vi "Dynamic Generation of Formula for Vtip.vi"(11 "Voltage (V)":T1={"Schedule"=enum."Constant", "Settings"=variant(dbl 10.0)}) -> (3 "Voltage (V) 2":T1={"Schedule"=enum."Constant", "Settings"=variant(dbl 10.0)})   [LabVIEW 2019]
uses:
  typedefs/Voltage - cluster.ctl
  typedefs/Schedule - enum.ctl
  typedefs/Schedule Types/Schedule--Formula.ctl
  <vilib>/gmath/NI_Gmath.lvlib
panel:
  out "error":i32
  in  "formula":string="1*(step(170-t)*cos(0.62831853071*t)+step(t-170)*cos(0.62831853071*(t-170))*(-1))"
  out "XY Graph":cluster{"X Values":dbl[], "Y Values":dbl[]}(graph)
  in  "Resolution (nm)":dbl=0.001
  in  "Length (nm)":dbl=340.0
  in  "OK":bool
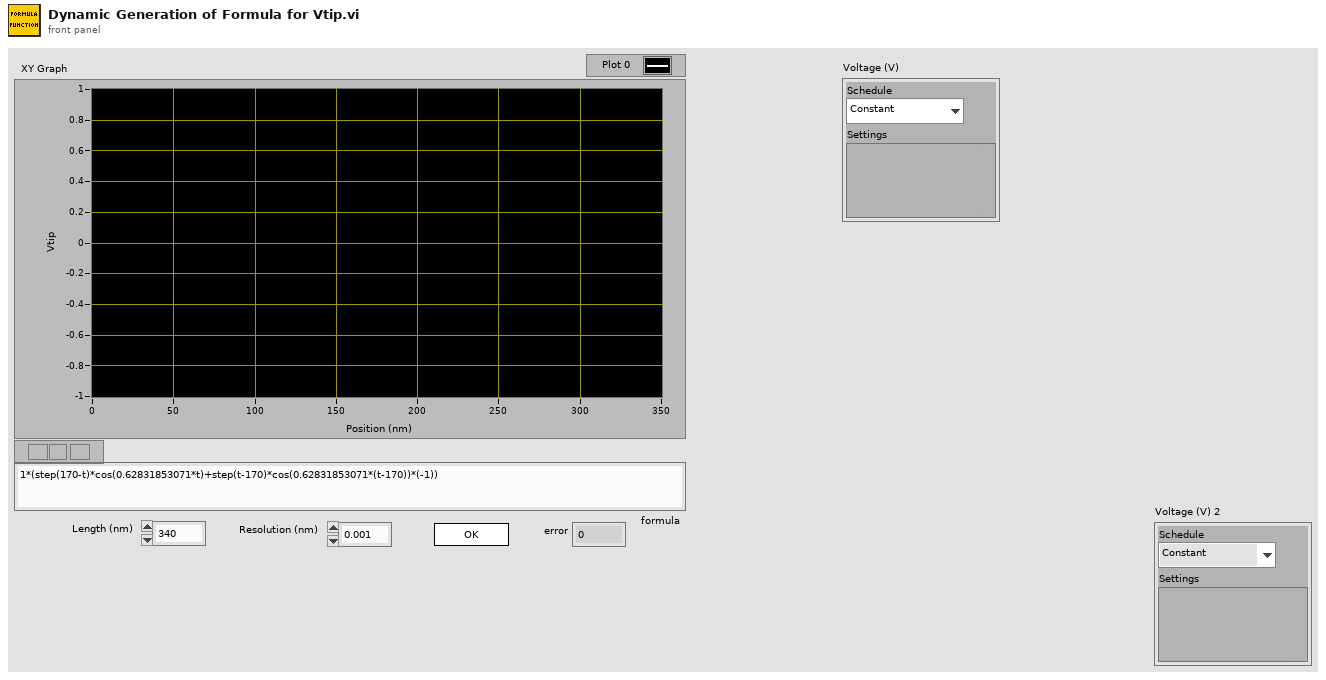
[diagram p1: front panel]
types:
  T1 = typedef "Voltage - cluster.ctl" = cluster{"Schedule":T2, "Settings":variant}
  T2 = typedef "Schedule - enum.ctl" = enum16{"Constant", "Ramp", "Fn. Generator", "Formula"}
  T3 = enum32{"invalid app kind", "Development System", "Run Time System", "Student Edition", "Embedded LabVIEW", "Evaluation", "Custom"}
  T4 = enum32{"Invalid", "Standard", "Closed", "Hidden", "Minimized", "Maximized"}
  T5 = typedef "Schedule--Formula.ctl" = cluster{"formula":string, "formula length (nm)":dbl, "formula resolution (nm)":dbl}
  T6 = cluster{"Core":cluster{"Current VI Reference":refnum<vi>, "Close Panel on Exit?":bool}, "Your Boolean data":bool, "Your string data":string, "# s":u32, "Voltage (V)":T1}
  T7 = cluster{"Current VI Reference":refnum<vi>, "Close Panel on Exit?":bool}
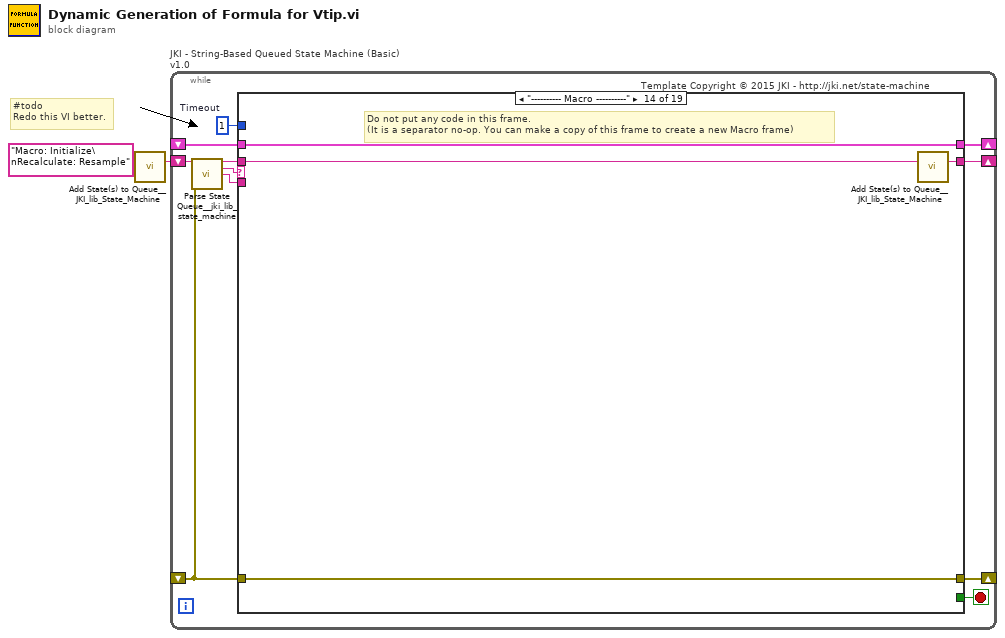
[diagram p0: block diagram]
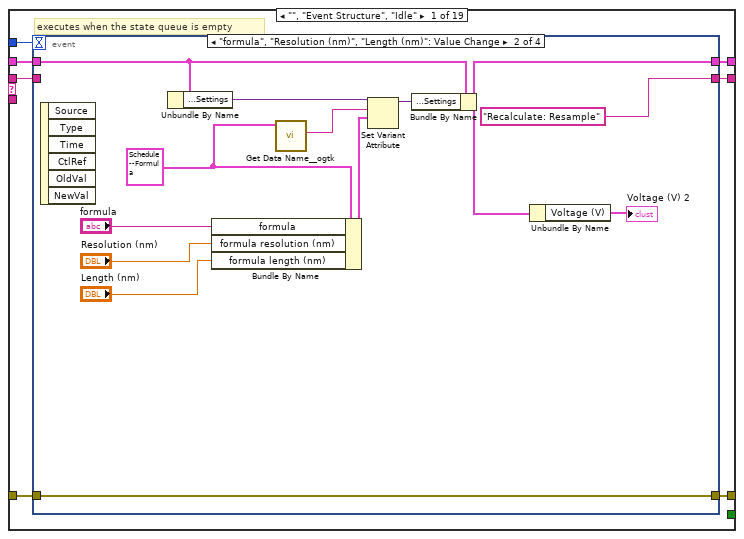
[diagram p2: hidden frame]
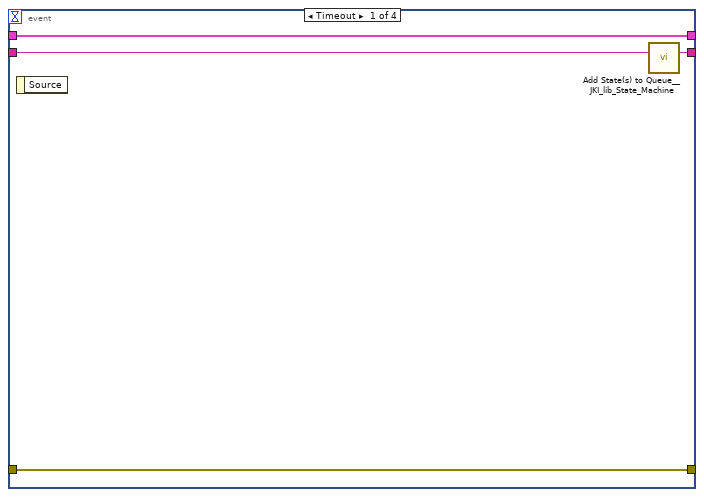
[diagram p3: hidden frame]
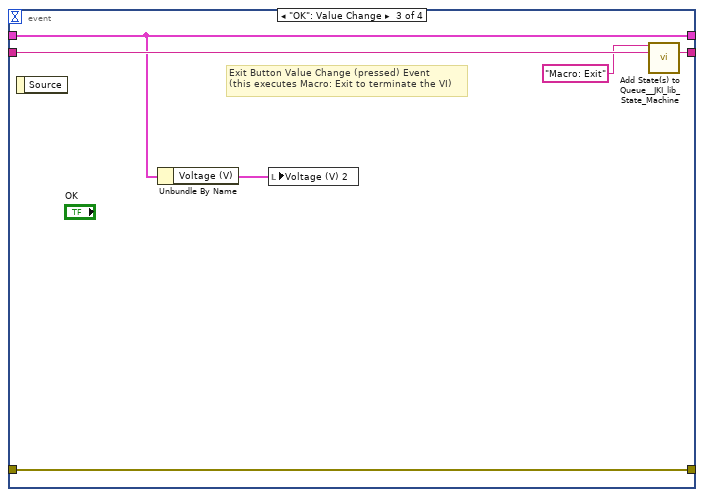
[diagram p4: hidden frame]
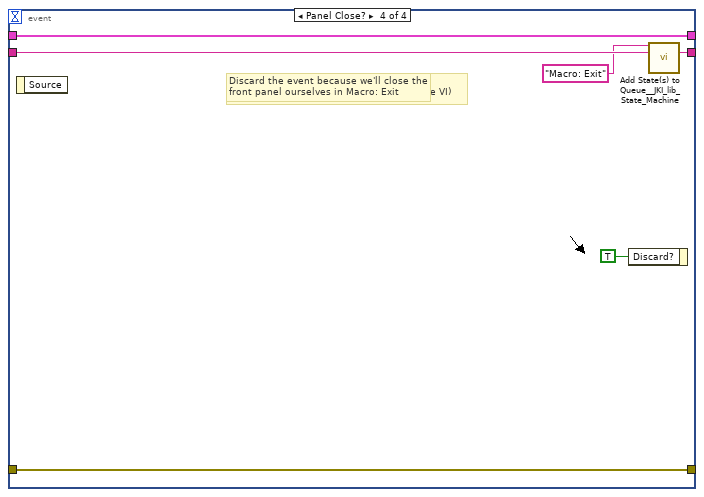
[diagram p5: hidden frame]
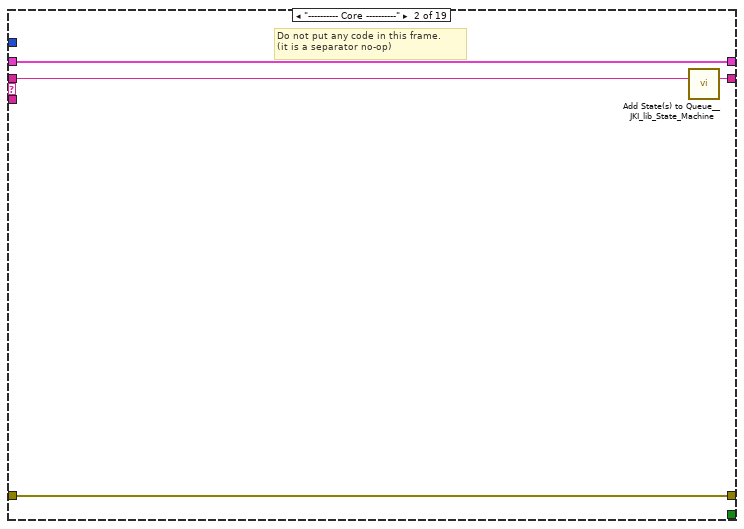
[diagram p6: hidden frame]
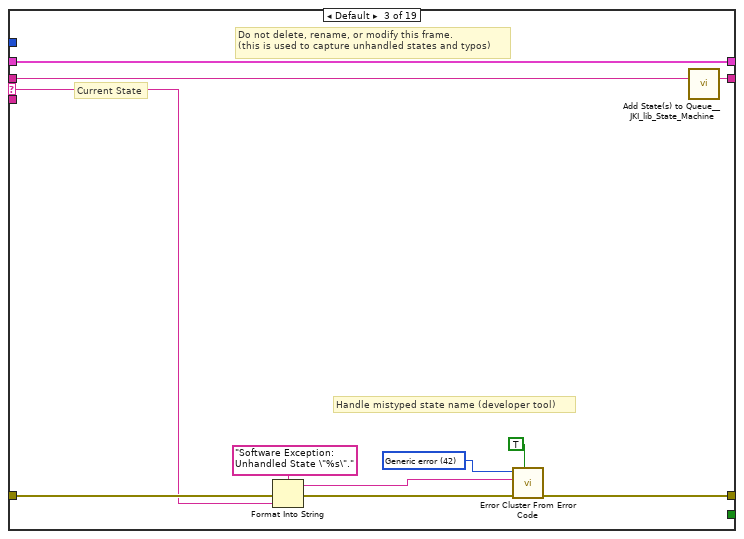
[diagram p7: hidden frame]
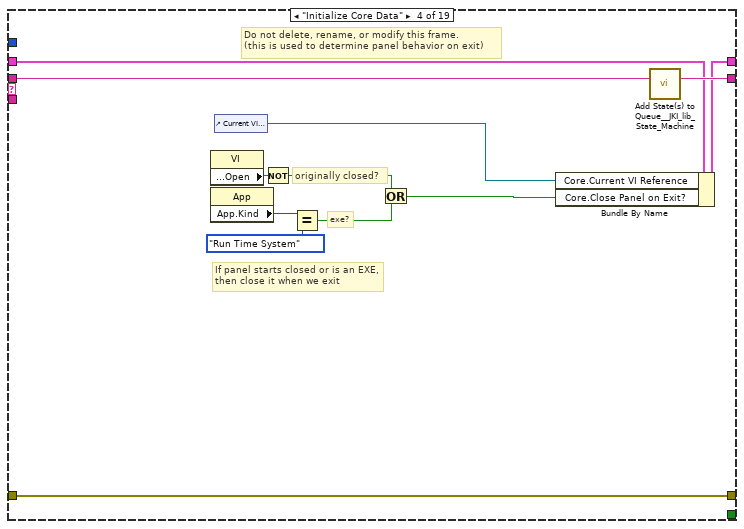
[diagram p8: hidden frame]
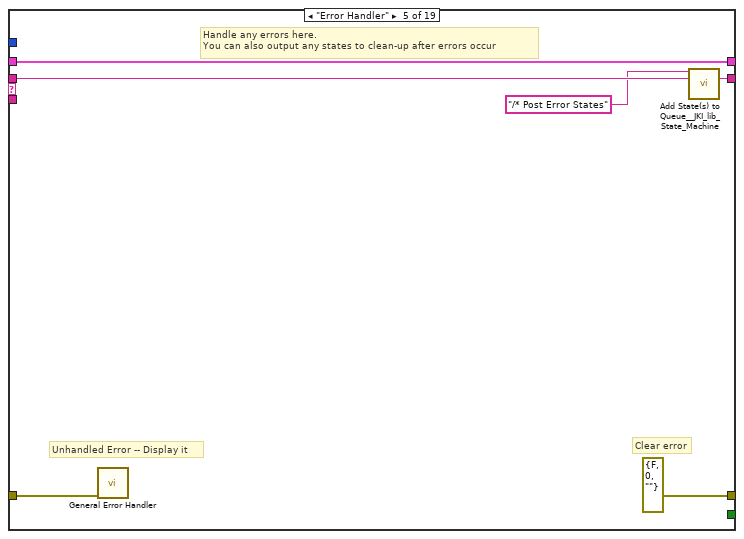
[diagram p9: hidden frame]
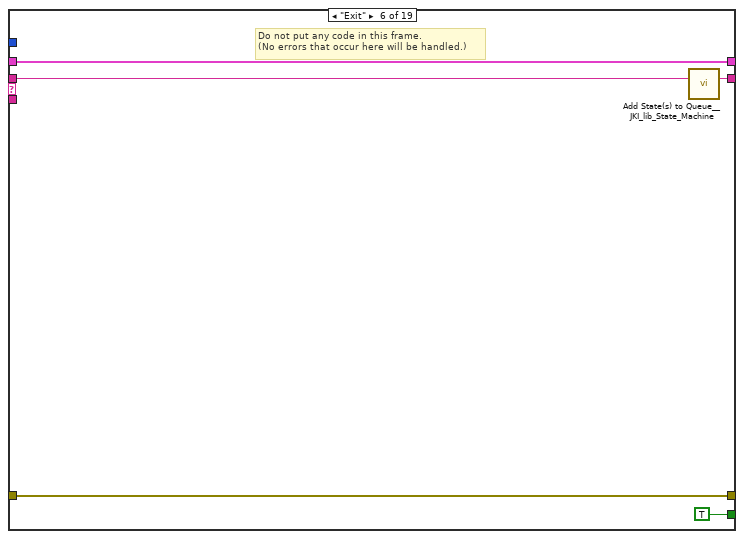
[diagram p10: hidden frame]
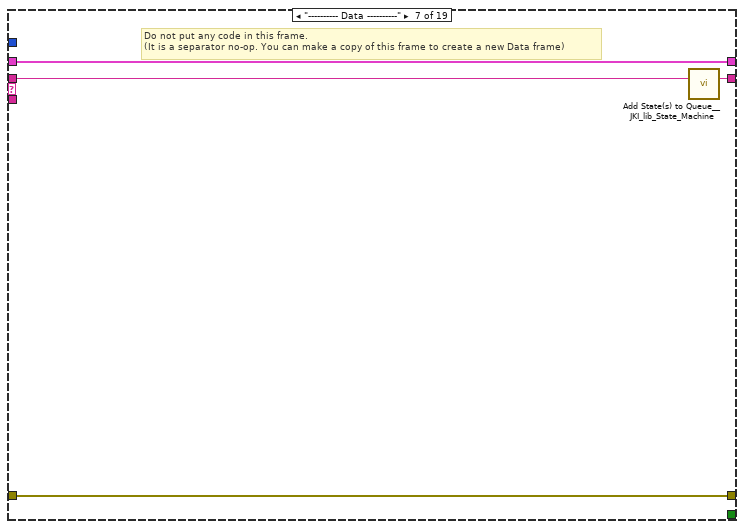
[diagram p11: hidden frame]
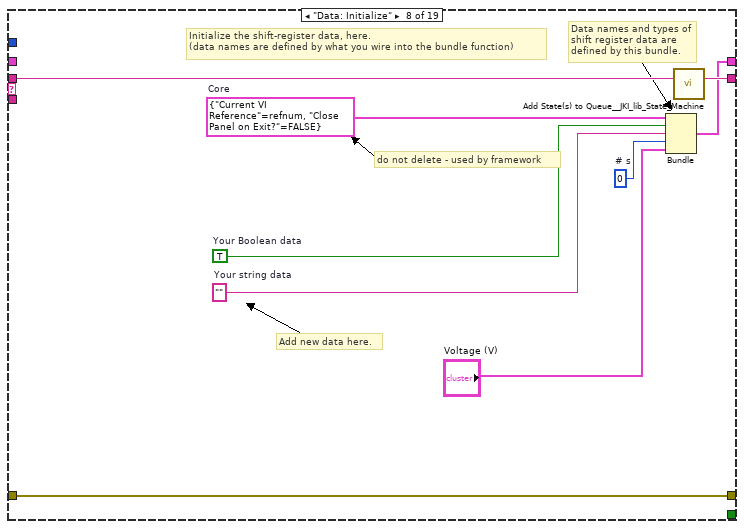
[diagram p12: hidden frame]
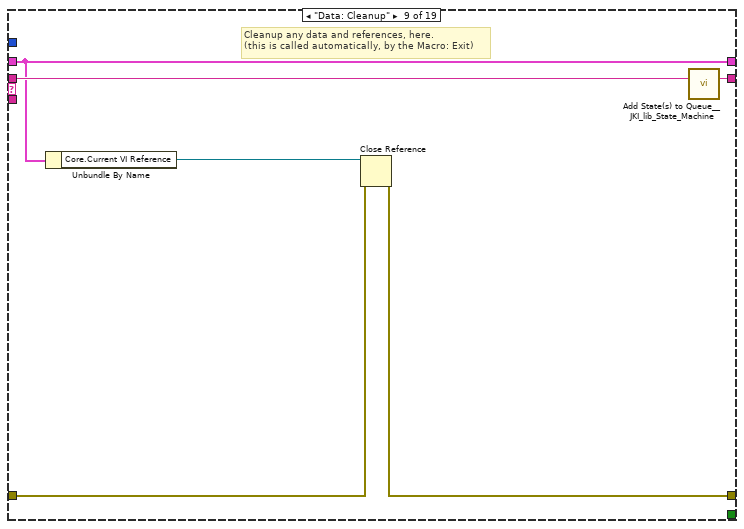
[diagram p13: hidden frame]
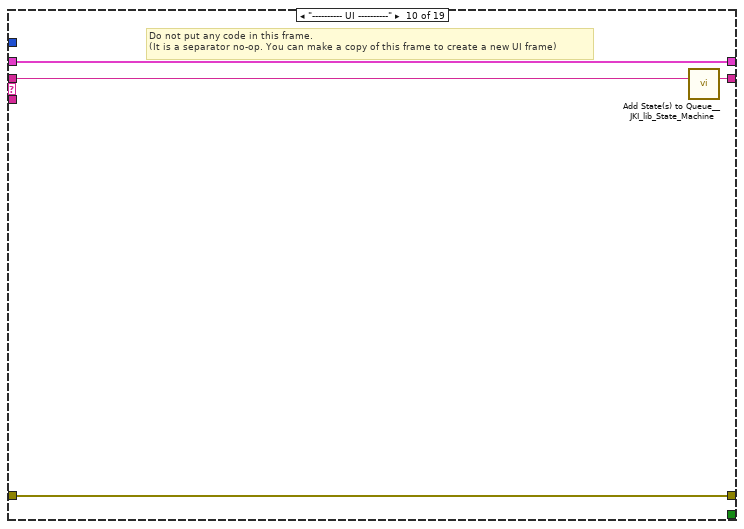
[diagram p14: hidden frame]
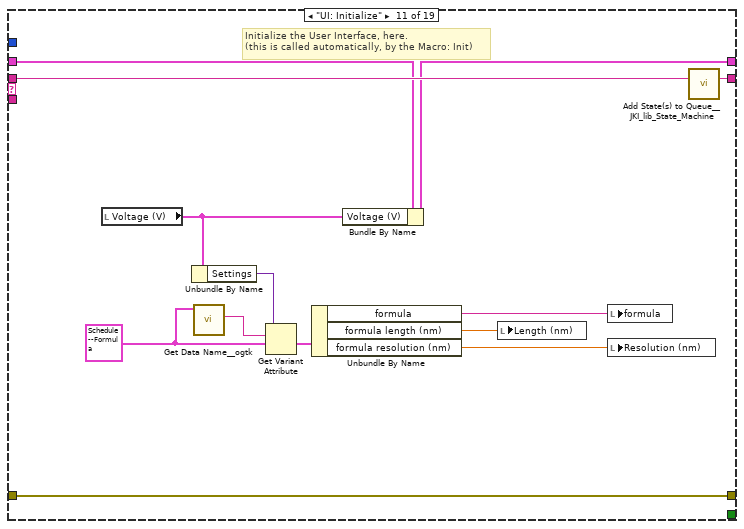
[diagram p15: hidden frame]
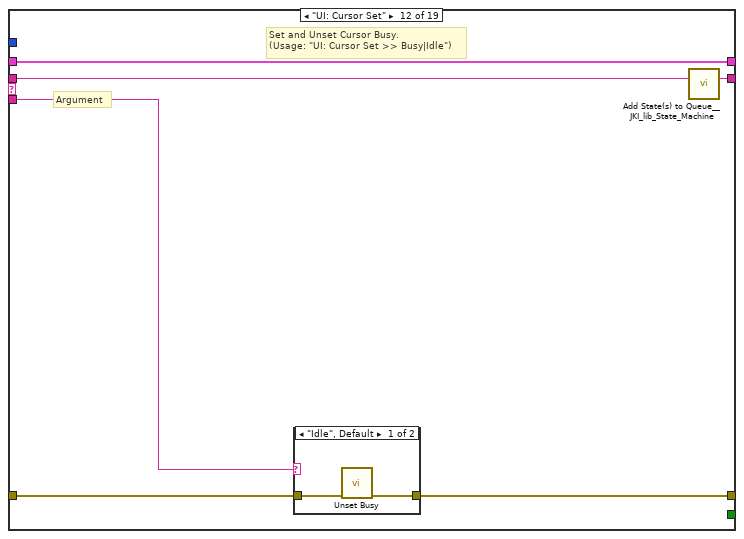
[diagram p16: hidden frame]
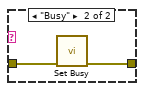
[diagram p17: hidden frame]
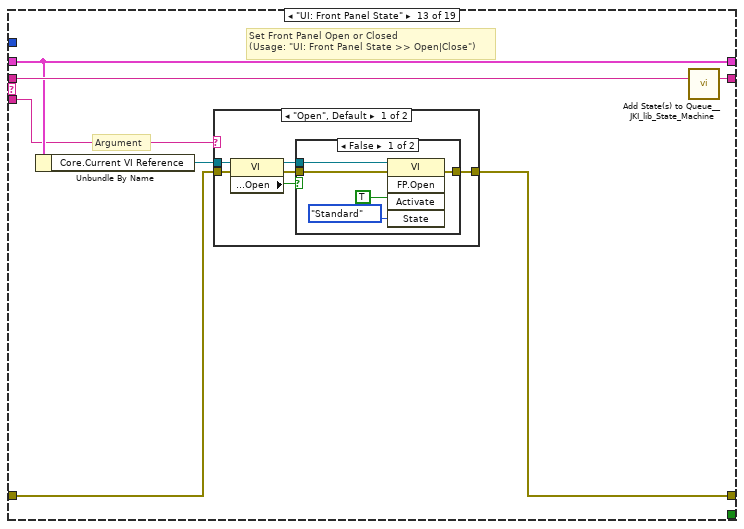
[diagram p18: hidden frame]
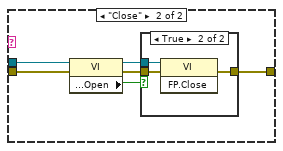
[diagram p20: hidden frame]
diagram:
  # "#todo\nRedo this VI better."
  n1 = call <vilib>:"Add State(s) to Queue__JKI_lib_State_Machine.vi"("State(s) in (\"\")"="Macro: Initialize\nRecalculate: Resample") -> ("States Out"=w2:string)  [unwired: 14 in]
  n2 = while "JKI - String-Based Queued State Machine (Basic) v1.0" {
    shift-right: [w6] -> _
    shift-left: _ -> [w5]
    shift-right: [w9] -> _
    shift-left: _ -> [w3]
    shift-right: [w8] -> _
    shift-left: w2 -> [w10]
    stop <- w7 stop-if-true
    w4 = 1  # Timeout
    # "Template Copyright © 2015 JKI - http://jki.net/state-machine"
    n3 = call <vilib>:"Parse State Queue__jki_lib_state_machine.vi"("State Queue"=w10, "Error In (no error)"=w3) -> ("Remaining States"=w12:string, "Current State"=w13:string, "Arguments"=w11:string)  [unwired: 11 in]
    n4 = case shown="\"---------- Macro ----------\"" w13 {
      selector: w13 -> [_ _ w54 _ _ _ _ _ _ _ _ _ _ _ _ _ _ _ _]
      tunnel: w12 -> [w20 w53 w58 w76 w82 w87 w91 w100 w106 w110 w123 w129 w140 w166 w171 w181 w185 w202 w206]
      tunnel: w11 -> [_ _ _ _ _ _ _ _ _ _ _ w124 w134 _ _ _ _ _ _]
      tunnel: w5 -> [w18 w50 w56 w67 w79 w85 w88 _ w101 w107 w120 w127 w136 w163 w168 w178 w182 w187 w203]
      tunnel: [w17 w51 w60 w73 errorcluster {"status"=FALSE, "code"=0, "source"=""} ("error out") w84 w89 w97 w102 w108 w121 w125 w137 w164 w169 w179 w183 w200 w204] -> w9
      tunnel: w3 -> [w16 w51 w59 w73 w78 w84 w89 w97 w103 w108 w121 w126 w138 w164 w169 w179 w183 w200 w204]
      tunnel: [w19 w52 w57 w75 w81 w86 w90 w99 w105 w109 w122 w128 w139 w165 w170 w180 w184 w201 w205] -> w8
      tunnel: [_ _ _ _ _ TRUE _ _ _ _ _ _ _ _ _ _ _ _ _] -> w7
      tunnel: [w15 w50 w56 w74 w79 w85 w88 w98 w101 w107 w111 w127 w136 w163 w168 w178 w182 w187 w203] -> w6
      tunnel: w4 -> [w14 _ _ _ _ _ _ _ _ _ _ _ _ _ _ _ _ _ _]
      frame "", "Event Structure", "Idle" {
        # "executes when the state queue is empty"
        n5 = event shown="[1] \"formula\", \"Resolution (nm)\", \"Length (nm)\": Value Change" {
          selector: _ -> [_ _ _ _]
          dyn-events: _ -> [_ _ _ _]
          timeout: w14 -> [_ _ _ _]
          tunnel: w20 -> [w24 _ w43 w49]
          tunnel: [w23 "Recalculate: Resample" w42 w48] -> w19
          tunnel: w18 -> [w21 w34 w39 w46]
          tunnel: [w22 w36 w41 w47] -> w17
          tunnel: w16 -> [w22 w36 w41 w47]
          tunnel: [w21 w31 w39 w46] -> w15
          event Timeout {
            n6 = event-data() -> ()  [unwired: 1 in, 1 out]
            n7 = call <vilib>:"Add State(s) to Queue__JKI_lib_State_Machine.vi"("State(s) in (\"\")"=w24) -> ("States Out"=w23:string)  [unwired: 14 in]
          }
          event "formula", "Resolution (nm)", "Length (nm)": Value Change {
            w26 = T5 {"formula"="1*(step(170-t)*cos(0.62831853071*t)+step(t-170)*cos(0.62831853071*(t-170))*(-1))", "formula length (nm)"=340.0, "formula resolution (nm)"=0.001} ("Formula")
            n8 = event-data() -> ()  [unwired: 1 in, 6 out]
            n9 = Unbundle By Name(w34) -> ("Voltage (V).Settings"=w33:variant)
            n10 = Bundle By Name(cluster=w26, "formula"="formula", "formula resolution (nm)"="Resolution (nm)", "formula length (nm)"="Length (nm)") -> (w27:T5)
            n11 = call <userlib>:"Get Data Name__ogtk.vi"("Data"=w26) -> ("Data Name"=w25:string)  [unwired: 8 in, 2 out]
            n12 = Set Variant Attribute(Variant=w33, name=w25, value=w27) -> (Variant out=w32:variant)  [unwired: 1 in, 2 out]
            n13 = Bundle By Name(cluster=w34, "Voltage (V).Settings"=w32) -> (w31:T6)
            n14 = Unbundle By Name(w31) -> ("Voltage (V)"=→"Voltage (V) 2":T1)
          }
          event "OK": Value Change {
            # "Exit Button Value Change (pressed) Event\n(this executes Macro: Exit to terminate the VI)"
            n15 = event-data() -> ()  [unwired: 1 in, 1 out]
            n16 = Unbundle By Name(w39) -> ("Voltage (V)"=w38:T1)
            n17 = local write "Voltage (V) 2"(w38) -> ()
            n18 = call <vilib>:"Add State(s) to Queue__JKI_lib_State_Machine.vi"("State(s) in Front (\"\")"="Macro: Exit", "State(s) in (\"\")"=w43) -> ("States Out"=w42:string)  [unwired: 13 in]
          }
          event Panel Close? {
            # "Discard the event because we'll close the front panel ourselves in Macro: Exit"
            # "Close Panel button (pressed) Event\n(this executes Macro: Exit to terminate the VI)"
            n19 = event-data() -> ()  [unwired: 1 in, 1 out]
            n20 = event-data("Discard?"=TRUE) -> ()  [unwired: 1 in, 1 out]
            n21 = call <vilib>:"Add State(s) to Queue__JKI_lib_State_Machine.vi"("State(s) in Front (\"\")"="Macro: Exit", "State(s) in (\"\")"=w49) -> ("States Out"=w48:string)  [unwired: 13 in]
          }
        }
      }
      frame "---------- Core ----------" {
        # "Do not put any code in this frame.\n(it is a separator no-op)"
        n22 = call <vilib>:"Add State(s) to Queue__JKI_lib_State_Machine.vi"("State(s) in (\"\")"=w53) -> ("States Out"=w52:string)  [unwired: 14 in]
      }
      frame Default {
        w63 = 42 items=["No error", "Argument error", "Memory is full", "Out of zone", "End of file", "File already open", "Generic file I/O error", "File not found", "File permission error", "Disk is full", "Duplicate path", "Too many files open", "System feature not enabled", "Resource file not found", "Cannot add resource", "Resource not found", "Image not found", "Image memory error", "Pen does not exist", "Config type invalid", "Config token not found", "Config parse error", "Config memory error", "Bad external code format", "Bad external code offset", "External code not present", "Null window", "Destroy window error", "Null menu", "Print aborted", "Bad print record", "Print driver error", "Windows error during printing", "Memory error during printing", "Print dialog error", "Generic print error", "Invalid device refnum", "Device not found", "Device parameter error", "Device unit error", "Cannot open device", "Device call aborted", "Generic error", "Cancelled by user", "Object ID too low", "Object ID too high", "Object not in heap", "Unknown heap", "Unknown object (invalid DefProc)", "Unknown object (DefProc not in table)", "Message out of range", "Invalid (null) method", "Unknown message", "Manager call not supported", "Bad address", "Network operation in progress", "Network operation timed out", "Connection is busy", "Network attribute not supported", "Network error", "Address in use", "System out of memory", "Connection aborted", "Connection refused", "Not connected", "Already connected", "Connection closed", "Initialization error (interapplication manager)", "Bad occurrence", "Wait on unbound occurrence handler", "Occurrence queue overflow", "Datalog type conflict", "Unused", "Unrecognized type (interapplication manager)", "Memory corrupt", "Failed to make temporary DLL", "Old CIN version", "Drag socket not found", "Failed to load drop-object", "Failed to register OLE object", "Failed to release OLE object", "Format specifier type mismatch", "Unknown format specifier", "Too few format specifiers", "Too many format specifiers", "Scan failed", "Newer CIN version", "Error converting to variant", "Runtime menu error", "Password tampered", "Variant attribute not found", "Incompatible variant data type", "Event data is not available", "Event Store is not present", "Occurrence is not found", "Event Queue is not created", "Event info is not available", "Refnum passed is NULL", "Error retrieving Class GUID", "Error retrieving CoClass GUID", "Error retrieving TypeLib GUID.", "Bad built application magic bytes.", "Specific driver is different from the specific driver associated with the Logical Name.", "There is no session opened to the class driver.", "Max Error", "MAX - Error with config objects", "MAX - Error loading configuration", "MAX - Group not supported"]
        # "Current State"
        # "Do not delete, rename, or modify this frame.\n(this is used to capture unhandled states and typos)"
        # "Handle mistyped state name (developer tool)"
        n23 = Format Into String(format string="Software Exception: Unhandled State \"%s\"." ("message"), error in=w59, w54) -> (resulting string=w62:string, error out=w61:errorcluster)  [unwired: 1 in]
        n24 = call <vilib>:"Error Cluster From Error Code.vi"("show call chain? (False)"=TRUE, "error in (no error)"=w61, "error message (\"\")"=w62, "error code (0)"=w63) -> ("error out"=w60:errorcluster)  [unwired: 5 in]
        n25 = call <vilib>:"Add State(s) to Queue__JKI_lib_State_Machine.vi"("State(s) in (\"\")"=w58) -> ("States Out"=w57:string)  [unwired: 14 in]
      }
      frame "Initialize Core Data" {
        # "Do not delete, rename, or modify this frame.\n(this is used to determine panel behavior on exit)"
        # "originally closed?"
        # "exe?"
        # "If panel starts closed or is an EXE, then close it when we exit"
        n26 = property class="VI"() -> ("Front Panel.Open"=w72:bool)  [unwired: 2 in, 2 out]
        n27 = property class="App"() -> ("App.Kind"=w71:T3)  [unwired: 2 in, 2 out]
        n28 = control-ref of="Current VI Reference"() -> (w65:refnum<vi>)
        n29 = Not(x=w72) -> (.not. x?=w69:bool)
        n30 = Equal?(x=w71, y=T3."Run Time System" ("Application:Kind")) -> (x = y?=w68:bool)
        n31 = Or(x=w69, y=w68) -> (x .or. y?=w66:bool)
        n32 = Bundle By Name(cluster=w67, "Core.Current VI Reference"=w65, "Core.Close Panel on Exit?"=w66) -> (w74:T6)
        n33 = call <vilib>:"Add State(s) to Queue__JKI_lib_State_Machine.vi"("State(s) in (\"\")"=w76) -> ("States Out"=w75:string)  [unwired: 14 in]
      }
      frame "Error Handler" {
        # "Unhandled Error -- Display it"
        # "Handle any errors here.\nYou can also output any states to clean-up after errors occur"
        # "Clear error"
        n34 = call <vilib>:"General Error Handler.vi"("error in (no error)"=w78) -> ()  [unwired: 10 in, 5 out]
        n35 = call <vilib>:"Add State(s) to Queue__JKI_lib_State_Machine.vi"("State(s) in Front (\"\")"="/* Post Error States", "State(s) in (\"\")"=w82) -> ("States Out"=w81:string)  [unwired: 13 in]
      }
      frame "Exit" {
        # "Do not put any code in this frame.\n(No errors that occur here will be handled.)"
        n36 = call <vilib>:"Add State(s) to Queue__JKI_lib_State_Machine.vi"("State(s) in (\"\")"=w87) -> ("States Out"=w86:string)  [unwired: 14 in]
      }
      frame "---------- Data ----------" {
        # "Do not put any code in this frame.\n(It is a separator no-op. You can make a copy of this frame to create a new Data frame)"
        n37 = call <vilib>:"Add State(s) to Queue__JKI_lib_State_Machine.vi"("State(s) in (\"\")"=w91) -> ("States Out"=w90:string)  [unwired: 14 in]
      }
      frame "Data: Initialize" {
        w93 = u32 0  # # s
        w94 = T7 {"Current VI Reference"=refnum, "Close Panel on Exit?"=FALSE}  # Core
        w96 = TRUE  # Your Boolean data
        w95 = ""  # Your string data
        # "do not delete - used by framework"
        # "Add new data here."
        # "Data names and types of shift register data are defined by this bundle."
        # "Initialize the shift-register data, here.\n(data names are defined by what you wire into the bundle function)"
        n38 = Bundle("Core"=w94, "Your Boolean data"=w96, "Your string data"=w95, "# s"=w93, "Voltage (V)"="Voltage (V)") -> (w98:T6)  [unwired: 1 in]
        n39 = call <vilib>:"Add State(s) to Queue__JKI_lib_State_Machine.vi"("State(s) in (\"\")"=w100) -> ("States Out"=w99:string)  [unwired: 14 in]
      }
      frame "Data: Cleanup" {
        # "Cleanup any data and references, here.\n(this is called automatically, by the Macro: Exit)"
        n40 = Unbundle By Name(w101) -> ("Core.Current VI Reference"=w104:refnum<vi>)
        n41 = Close Reference(reference=w104, error in (no error)=w103) -> (error out=w102:errorcluster)
        n42 = call <vilib>:"Add State(s) to Queue__JKI_lib_State_Machine.vi"("State(s) in (\"\")"=w106) -> ("States Out"=w105:string)  [unwired: 14 in]
      }
      frame "---------- UI ----------" {
        # "Do not put any code in this frame.\n(It is a separator no-op. You can make a copy of this frame to create a new UI frame)"
        n43 = call <vilib>:"Add State(s) to Queue__JKI_lib_State_Machine.vi"("State(s) in (\"\")"=w110) -> ("States Out"=w109:string)  [unwired: 14 in]
      }
      frame "UI: Initialize" {
        w119 = T5 {"formula"="1*(step(170-t)*cos(0.62831853071*t)+step(t-170)*cos(0.62831853071*(t-170))*(-1))", "formula length (nm)"=340.0, "formula resolution (nm)"=0.001} ("Formula")
        # "Initialize the User Interface, here.\n(this is called automatically, by the Macro: Init)"
        n44 = local read "Voltage (V)"() -> (w114:T1)
        n45 = Unbundle By Name(w114) -> ("Settings"=w113:variant)
        n46 = call <userlib>:"Get Data Name__ogtk.vi"("Data"=w119) -> ("Data Name"=w118:string)  [unwired: 8 in, 2 out]
        n47 = Get Variant Attribute(Variant=w113, name=w118, default value (empty Variant)=w119) -> (value=w117:T5)  [unwired: 1 in, 3 out]
        n48 = Unbundle By Name(w117) -> ("formula"=w112:string, "formula length (nm)"=w116:dbl, "formula resolution (nm)"=w115:dbl)
        n49 = Bundle By Name(cluster=w120, "Voltage (V)"=w114) -> (w111:T6)
        n50 = local write "Length (nm)"(w116) -> ()
        n51 = local write "formula"(w112) -> ()
        n52 = local write "Resolution (nm)"(w115) -> ()
        n53 = call <vilib>:"Add State(s) to Queue__JKI_lib_State_Machine.vi"("State(s) in (\"\")"=w123) -> ("States Out"=w122:string)  [unwired: 14 in]
      }
      frame "UI: Cursor Set" {
        # "Argument"
        # "Set and Unset Cursor Busy.\n(Usage: \"UI: Cursor Set >> Busy|Idle\")"
        n54 = case shown="\"Idle\", Default" w124 {
          tunnel: w126 -> [w131 w133]
          tunnel: [w130 w132] -> w125
          frame "Idle", Default {
            n55 = call <vilib>:"Unset Busy.vi"("error in (no error)"=w131) -> ("error out"=w130:errorcluster)  [unwired: 10 in]
          }
          frame "Busy" {
            n56 = call <vilib>:"Set Busy.vi"("error in (no error)"=w133) -> ("error out"=w132:errorcluster)  [unwired: 9 in, 1 out]
          }
        }
        n57 = call <vilib>:"Add State(s) to Queue__JKI_lib_State_Machine.vi"("State(s) in (\"\")"=w129) -> ("States Out"=w128:string)  [unwired: 14 in]
      }
      frame "UI: Front Panel State" {
        # "Argument"
        # "Set Front Panel Open or Closed\n(Usage: \"UI: Front Panel State >> Open|Close\")"
        n58 = Unbundle By Name(w136) -> ("Core.Current VI Reference"=w135:refnum<vi>)
        n59 = case shown="\"Open\", Default" w134 {
          tunnel: w138 -> [w144 w157]
          tunnel: [w146 w158] -> w137
          tunnel: w135 -> [w145 w155]
          frame "Open", Default {
            n60 = property class="VI"(reference=w145, error in=w144) -> (reference out=w142:refnum<vi>, error out=w143:errorcluster, "Front Panel.Open"=w141:bool)
            n61 = case shown="False" w141 {
              tunnel: [w149 w152] -> w146
              tunnel: w143 -> [w148 w152]
              tunnel: w142 -> [w147 _]
              frame False {
                n62 = invoke class="VI" method="FP.Open"(reference=w147, error in=w148, "Activate"=TRUE, "State"=T4."Standard") -> (error out=w149:errorcluster)  [unwired: 1 in, 4 out]
              }
              frame True {
              }
            }
          }
          frame "Close" {
            n63 = property class="VI"(reference=w155, error in=w157) -> (reference out=w154:refnum<vi>, error out=w156:errorcluster, "Front Panel.Open"=w153:bool)
            n64 = case shown="True" w153 {
              tunnel: [w159 w162] -> w158
              tunnel: w156 -> [w159 w161]
              tunnel: w154 -> [_ w160]
              frame False {
              }
              frame True {
                n65 = invoke class="VI" method="FP.Close"(reference=w160, error in=w161) -> (error out=w162:errorcluster)  [unwired: 1 in, 2 out]
              }
            }
          }
        }
        n66 = call <vilib>:"Add State(s) to Queue__JKI_lib_State_Machine.vi"("State(s) in (\"\")"=w140) -> ("States Out"=w139:string)  [unwired: 14 in]
      }
      frame "---------- Macro ----------" {
        # "Do not put any code in this frame.\n(It is a separator no-op. You can make a copy of this frame to create a new Macro frame)"
        n67 = call <vilib>:"Add State(s) to Queue__JKI_lib_State_Machine.vi"("State(s) in (\"\")"=w166) -> ("States Out"=w165:string)  [unwired: 14 in]
      }
      frame "Macro: Initialize" {
        w167 = "Data: Initialize\nInitialize Core Data\nUI: Initialize\nUI: Front Panel State >> Open"  # Data: Initialize Initialize Core Data UI: Initialize UI: Front Panel State >> Open
        # "Initialization Macro\n(This is called once, when the VI starts)"
        n68 = call <vilib>:"Add State(s) to Queue__JKI_lib_State_Machine.vi"("State(s) in Front (\"\")"=w167, "State(s) in (\"\")"=w171) -> ("States Out"=w170:string)  [unwired: 13 in]
      }
      frame "Macro: Exit" {
        # "Exit Macro\n(This is called once, when the VI exits)"
        n69 = Unbundle By Name(w178) -> ("Core.Close Panel on Exit?"=w177:bool)
        n70 = Select(t="UI: Front Panel State >> Close", s=w177, f="") -> (s? t:f=w174:string)
        n71 = call <vilib>:"Add State(s) to Queue__JKI_lib_State_Machine.vi"("State(s) in (\"\")"=w174, "State(s) at Back (\"\")"="Data: Cleanup\nExit") -> ("States Out"=w172:string)  [unwired: 13 in]
        n72 = call <vilib>:"Add State(s) to Queue__JKI_lib_State_Machine.vi"("State(s) in Front (\"\")"=w172, "State(s) in (\"\")"=w181) -> ("States Out"=w180:string)  [unwired: 13 in]
      }
      frame "---------- Recalculate ----------" {
        # "Template Separator\n(You can make a copy of, or modify, this frame)"
        n73 = call <vilib>:"Add State(s) to Queue__JKI_lib_State_Machine.vi"("State(s) in (\"\")"=w185) -> ("States Out"=w184:string)  [unwired: 14 in]
      }
      frame "Recalculate: Resample" {
        w192 = T5 {"formula"="1*(step(170-t)*cos(0.62831853071*t)+step(t-170)*cos(0.62831853071*(t-170))*(-1))", "formula length (nm)"=340.0, "formula resolution (nm)"=0.001} ("Formula")
        # "Your code here.\n(You can make a copy of, or modify, this frame)"
        n74 = call <userlib>:"Get Data Name__ogtk.vi"("Data"=w192) -> ("Data Name"=w186:string)  [unwired: 8 in, 2 out]
        n75 = Unbundle By Name(w187) -> ("Voltage (V).Settings"=w193:variant)
        n76 = Get Variant Attribute(Variant=w193, name=w186, default value (empty Variant)=w192) -> (value=w191:T5)  [unwired: 1 in, 3 out]
        n77 = Unbundle By Name(w191) -> ("formula length (nm)"=w194:dbl, "formula resolution (nm)"=w195:dbl, "formula"=w188:string)
        n78 = Divide(x=w194, y=w195) -> (x/y=w197:dbl)
        n79 = call <vilib>:"Eval y=f(x).vi"("formula"=w188, "end"=w194, "start"=0.0, "number of points"=w197) -> ("error"=→"error":i32, "Y Values"=w198:dbl[], "X Values"=w199:dbl[])  [unwired: 1 out]
        n80 = Bundle("X Values"=w199, "Y Values"=w198) -> (→"XY Graph":cluster{"X Values":dbl[], "Y Values":dbl[]})  [unwired: 1 in]
        n81 = call <vilib>:"Add State(s) to Queue__JKI_lib_State_Machine.vi"("State(s) in (\"\")"=w202) -> ("States Out"=w201:string)  [unwired: 14 in]
      }
      frame "New Category: 2" {
        # "Your code here.\n(You can make a copy of, or modify, this frame)"
        n82 = call <vilib>:"Add State(s) to Queue__JKI_lib_State_Machine.vi"("State(s) in (\"\")"=w206) -> ("States Out"=w205:string)  [unwired: 14 in]
      }
    }
  }
